vi "FFT_based_prediction_SNR.vi"() -> ()   [LabVIEW 2020]
uses:
  <vilib>/Utility/file.llb/Read Delimited Spreadsheet (DBL).vi
  <vilib>/measure/mascope.llb/Cycle Average and RMS 1 chan.vi
  <vilib>/measure/NI_MAPro.lvlib
panel:
  out "error cycle RMS":dbl format="%.2g"
  out "pred cycle RMS":dbl format="%.2g"
  out "truth cycle RMS":dbl format="%.2g"
  out "Input vs prediction (zoomed)":dbl[][](graph)
  out "truth vs prediction vs error":dbl[][](graph)
  out "Input vs prediction":dbl[][](graph)
  out "Time vs Acceleration ( Input learning length)":cluster{dbl[], dbl[]}[](graph)
  out "truth vs prediction":dbl[][](graph)
  out "Spectrum plot 2":cluster{i32, dbl, "spectrum out":dbl[]}(graph)
  out "Frequency Interval: delta(f) 2":dbl
  out "xf (frequency) 2":dbl[](array[numeric])
  out "size(s) 2":i32
  out "df (Hz) 2":dbl
  out "ploted signal from each selected frequency 2":dbl[][](graph)
  out "phase 3":dbl[](array[numeric])
  out "magnitude 3":dbl[](array[numeric])
  out "Time vs Acceleration graph(whole data)":cluster{"all rows":dbl[], "all rows":dbl[]}(graph)
  out "Acceleration 2":dbl[](array[numeric])
  out "time 2":dbl[](array[numeric])
  out "array w/ subset deleted 2":dbl[][](array[numeric])
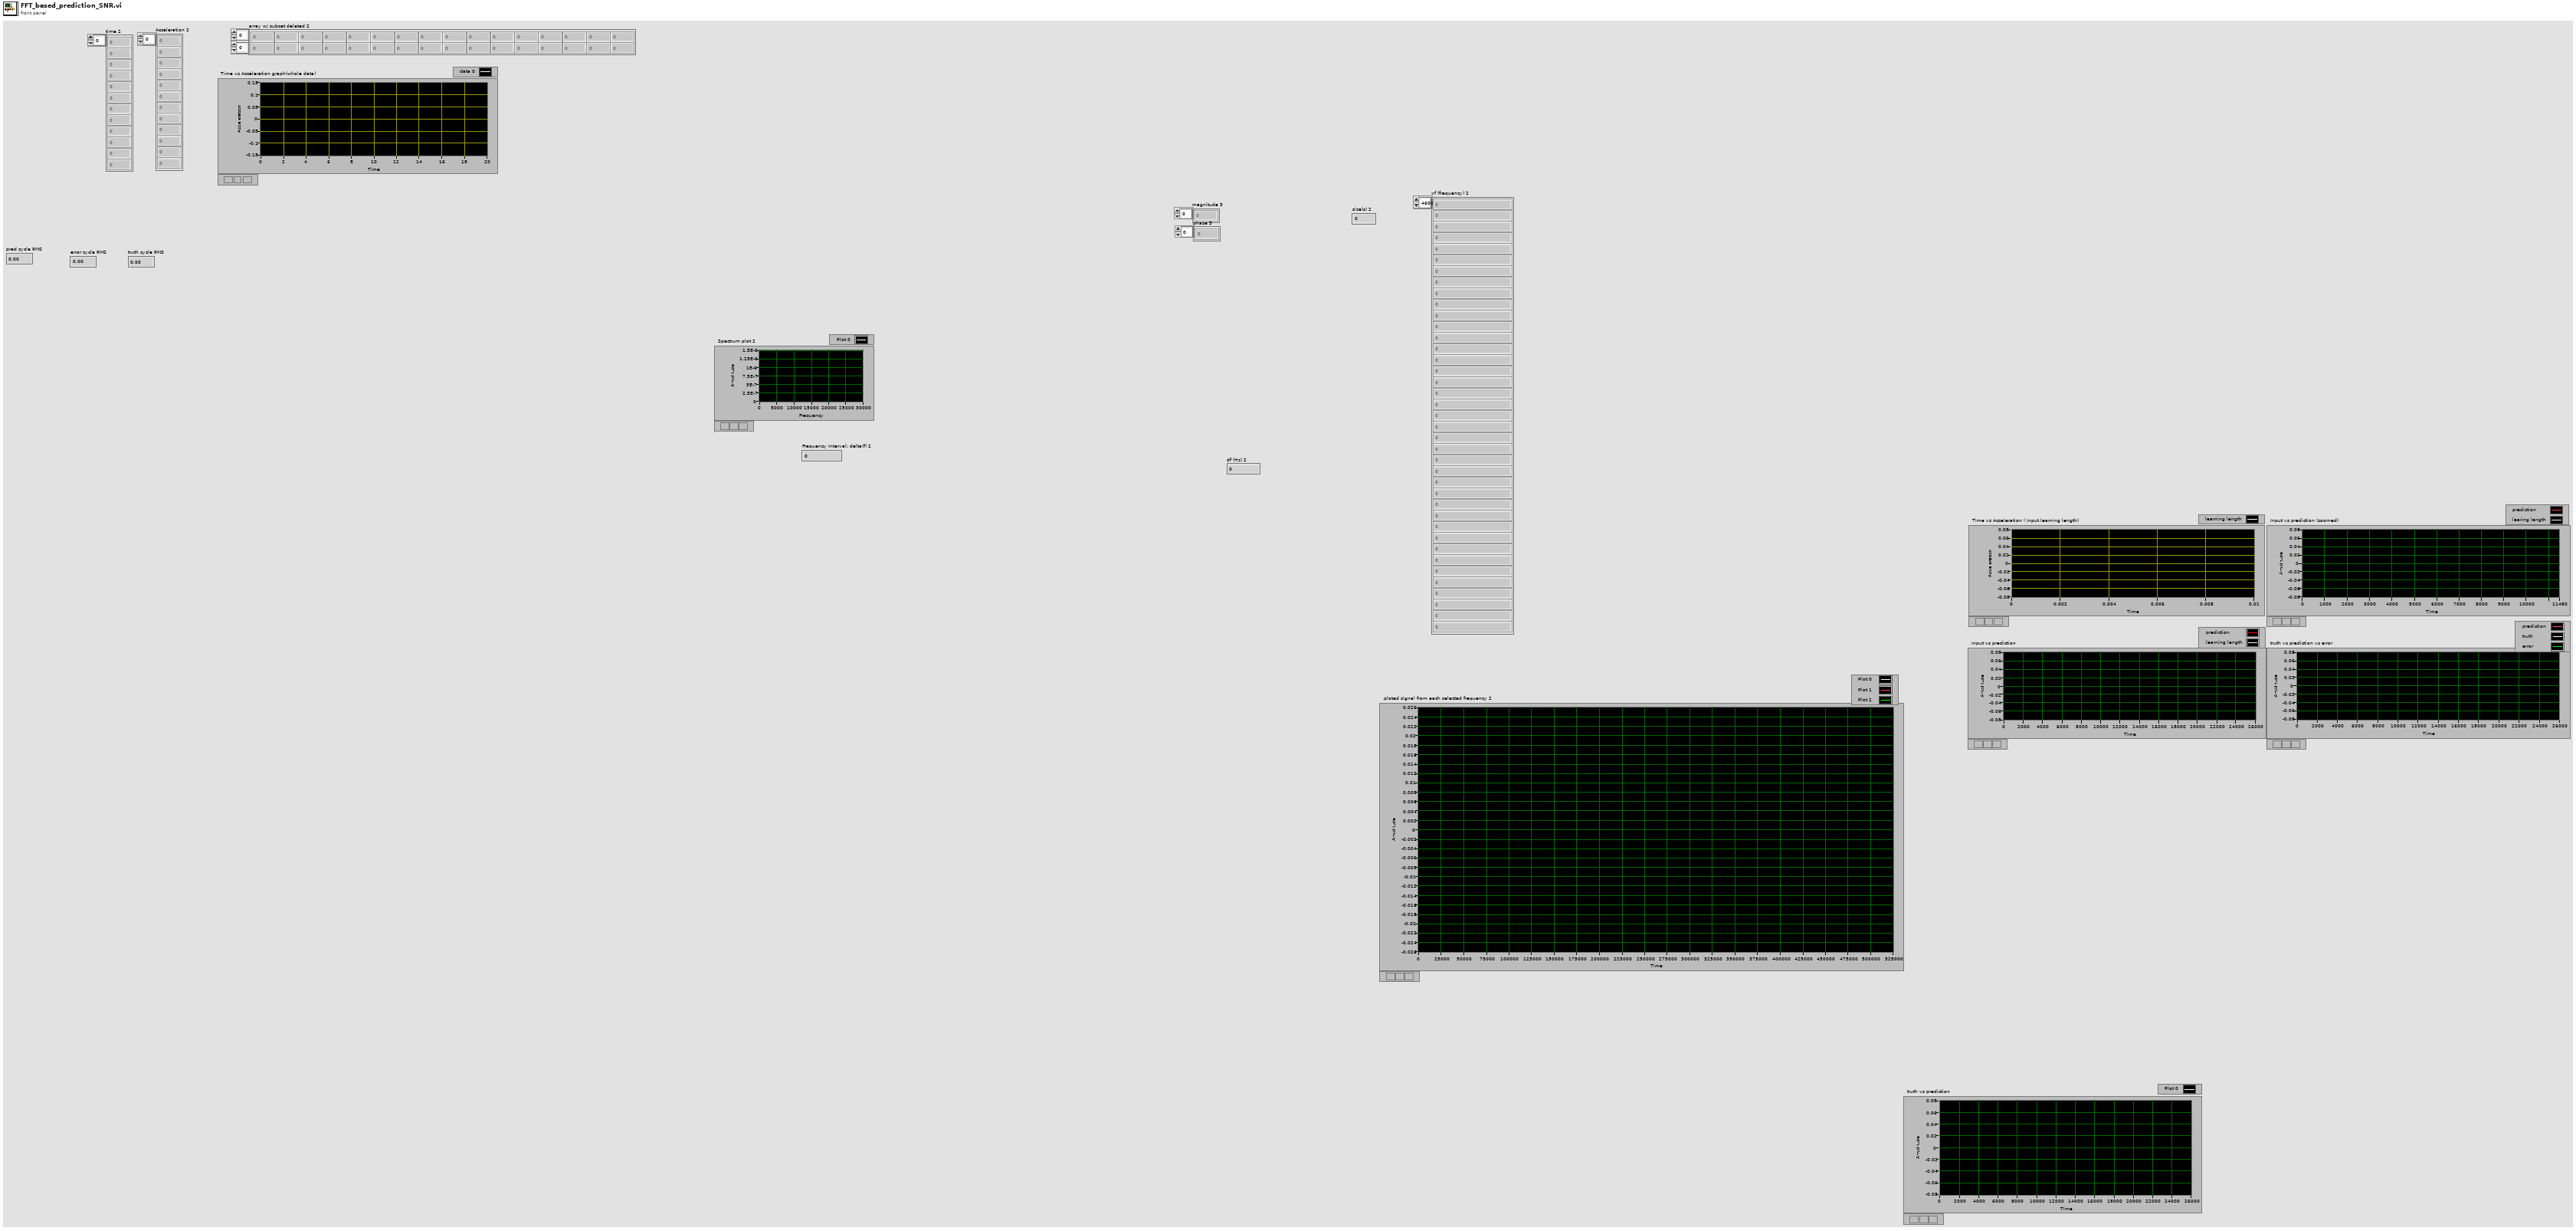
[diagram p1: front panel]
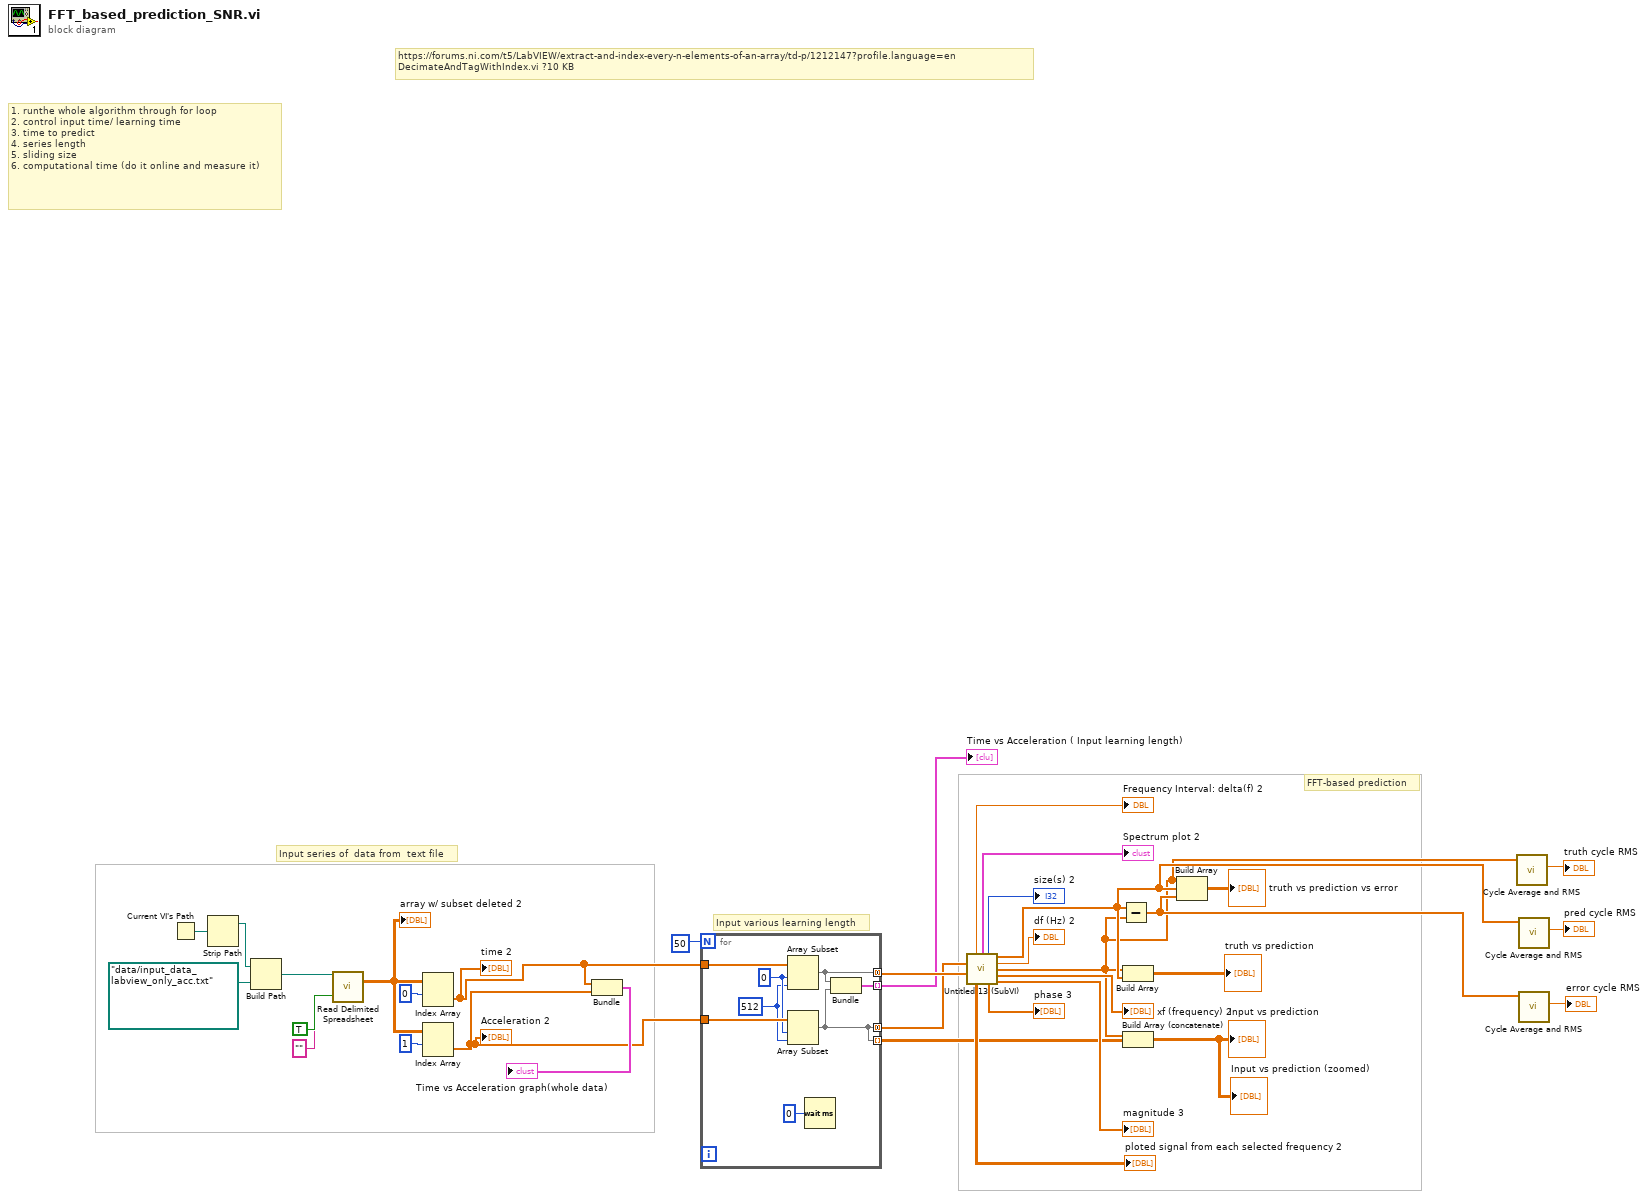
[diagram p0: block diagram]
diagram:
  # "Input series of  data from  text file"
  # "Input various learning length"
  # "FFT-based prediction"
  # "1. runthe whole algorithm through for loop \n2. control input time/ learning time\n3. time to predict\n4. series length\n5. sliding size\n6. computational time (do it online and measure it)"
  # "https://forums.ni.com/t5/LabVIEW/extract-and-index-every-n-elements-of-an-array/td-p/1212147?profile.language=en\nDecimateAndTagWithIndex.vi ?10 KB"
  n1 = Current VI's Path() -> (path=w32:path)
  n2 = Strip Path(path=w32) -> (stripped path=w33:path)  [unwired: 1 out]
  n3 = Build Path(base path=w33, name or relative path=path "data/input_data_labview_only_acc.txt") -> (appended path=w34:path)
  n4 = call-poly <vilib>:"Read Delimited Spreadsheet.vi"("file path (dialog if empty)"=w34, "transpose? (F)"=TRUE, "delimiter (\\t)"="" ("delimiter (\\t)")) -> ("all rows"=w31:dbl[][])  [unwired: 7 in, 5 out]
  "array w/ subset deleted 2" <- w31
  n5 = Index Array(array=w31, index (row)=0) -> (element=w16:dbl[])  [unwired: 1 in]
  "time 2" <- w16
  n6 = Index Array(array=w31, index (row)=1) -> (element=w1:dbl[])  [unwired: 1 in]
  "Acceleration 2" <- w1
  n7 = Bundle("all rows"=w16, "all rows"=w1) -> (→"Time vs Acceleration graph(whole data)":cluster{"all rows":dbl[], "all rows":dbl[]})  [unwired: 1 in]
  n8 = for {
    N: 50 -> [_]
    tunnel: w16 -> [w42]
    tunnel: [w39] -> w14 mode=concatenating
    tunnel: w1 -> [w41]
    tunnel: [w37] -> w13 mode=concatenating
    tunnel: [w38] -> w12 mode=indexing
    tunnel: [w37] -> w11 mode=indexing
    w40 = 0
    w36 = 512 ("length")
    n9 = Array Subset(array=w42, index=w40, length=w36) -> (w39:dbl[])
    n10 = Array Subset(array=w41, index=w40, length=w36) -> (w37:dbl[])
    n11 = Wait (ms)(milliseconds to wait=u32 0) -> ()  [unwired: 1 out]
    n12 = Bundle(w39, w37) -> (w38:cluster{dbl[], dbl[]})  [unwired: 1 in]
  }
  "Time vs Acceleration ( Input learning length)" <- w12
  n13 = call "Untitled 13 (SubVI).vi"("time"=w14, "acceleration"=w13) -> ("Frequency Interval: delta(f)"=→"Frequency Interval: delta(f) 2":dbl, "Spectrum plot"=→"Spectrum plot 2":cluster{i32, dbl, "spectrum out":dbl[]}, "size(s)"=→"size(s) 2":i32, "all rows"=w3:dbl[], "df (Hz)"=→"df (Hz) 2":dbl, "Array"=w2:dbl[], "xf (frequency)"=→"xf (frequency) 2":dbl[], "ploted signal from each selected frequency"=→"ploted signal from each selected frequency 2":dbl[][], "phase 2"=→"phase 3":dbl[], "magnitude 2"=→"magnitude 3":dbl[])  [unwired: 4 in]
  n14 = Subtract(x=w3, y=w2) -> (x-y=w4:dbl[])
  n15 = Build Array(w2, w3) -> (→"truth vs prediction":dbl[][])
  n16 = Build Array (concatenate)(w2, w11) -> (→"Input vs prediction" →"Input vs prediction (zoomed)":dbl[][])
  n17 = Build Array(w2, w3, w4) -> (→"truth vs prediction vs error":dbl[][])
  n18 = call-poly <vilib>:"Cycle Average and RMS.vi"("signal in"=w2) -> ("cycle RMS"=→"truth cycle RMS":dbl)  [unwired: 7 in, 3 out]
  n19 = call-poly <vilib>:"Cycle Average and RMS.vi"("signal in"=w3) -> ("cycle RMS"=→"pred cycle RMS":dbl)  [unwired: 7 in, 3 out]
  n20 = call-poly <vilib>:"Cycle Average and RMS.vi"("signal in"=w4) -> ("cycle RMS"=→"error cycle RMS":dbl)  [unwired: 7 in, 3 out]
